vi "find_best_fit.vi"(8 "error in (no error)":errorcluster, 10 "value to be found":dbl, 11 "search space":dbl[](array[numeric])) -> (0 "error out":errorcluster, 2 "indices of fits":i32[](array[numeric]), 3 "index of best match":i32)   [LabVIEW 2010]
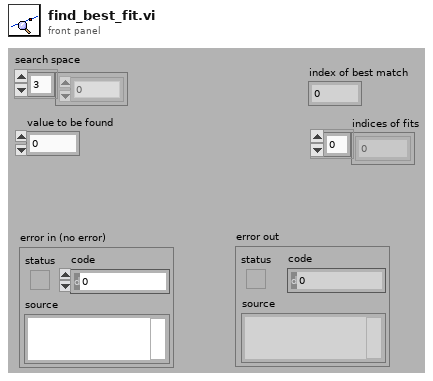
[diagram p1: front panel]
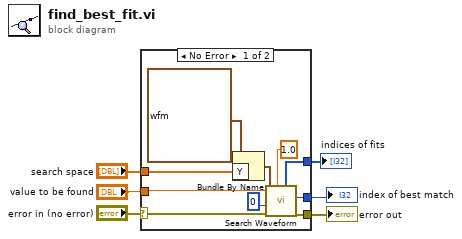
[diagram p0: block diagram]
diagram:
  n1 = case shown="No Error" "error in (no error)" {
    selector: "error in (no error)" -> [w12 w17]
    tunnel: [w16 w17] -> w6
    tunnel: "search space" -> [w14 _]
    tunnel: "value to be found" -> [w9 _]
    tunnel: [w11 _] -> w2
    tunnel: [w7 _] -> w1
    frame No Error {
      n2 = Bundle By Name(cluster=waveform(dbl) {"t0"=timestamp(0 s since 1904-01-01), "dt"=1.0, "Y"=[]} ("waveform in"), "Y"=w14) -> (w13:waveform(dbl))
      n3 = call <vilib>:"Search Waveform.vi"("tolerance (%)"=1.0, "error in (no error)"=w12, "start index"=0, "value"=w9, "waveform in"=w13) -> ("error out"=w16:errorcluster, "index of best fit"=w11:i32, "indices of fits"=w7:i32[])  [unwired: 1 in, 3 out]
    }
    frame Error {
    }
  }
  "error out" <- w6
  "index of best match" <- w2
  "indices of fits" <- w1
